vi "File Page - Set Start Trigger.vi"(7 "File Ctl Refs":T3, 8 "error in (no error)":errorcluster, 10 "Start Trigger":T1, 11 "Item Ref in":T2 format="%.0x") -> (0 "error out":errorcluster)   [LabVIEW 2015, in "Waveform Data Logger System Explorer.lvlib"]
uses:
  Waveform Data Logger System Explorer.lvlib
  Types/File Ctl Refs.ctl
  Types/File - Spec Ctl Refs.ctl
  Types/File - Wfm Ctl Refs.ctl
  Types/File - Settings Ctl Refs.ctl
  Shared/Classes/Log File Specifications/Log File Specification/File Conflict Operation.ctl
  Types/File - Start Trig Ctl Refs.ctl
  Shared/Types/Start Trigger.ctl
  Shared/Types/Default Trigger.ctl
  Shared/Types/Digital Trigger.ctl
  Shared/Types/Analog Trigger.ctl
  Shared/Types/In Range Trigger.ctl
  Shared/Types/Value Change Trigger.ctl
  Shared/Types/Boolean Trigger.ctl
  Types/Single Node Browser Data.ctl
  <vilib>/NI Veristand/UI Controls/Single Node Browser/Single Node Browser Ref.ctl
  NationalInstruments.VeriStand.SystemStorageUI
  <vilib>/NI Veristand/UI Controls/Single Node Browser/Callback Type.ctl
  <vilib>/NI Veristand/UI Controls/Single Node Browser/Net Event Data.ctl
  <vilib>/NI Veristand/UI Controls/Single Node Browser/Net Event.ctl
  Types/File - Stop Trig Ctl Refs.ctl
  Shared/Types/Stop Trigger.ctl
  Types/File - Advanced Ctl Refs.ctl
  Types/Log Timestamps.ctl
  <vilib>/NI Veristand/Custom Device API/Custom Device Item Ref.ctl
  NationalInstruments.VeriStand.SystemStorage
  Shared/Globals/Property Strings.vi
  <vilib>/NI Veristand/Custom Device API/Set Item Property (U16).vi
  <vilib>/NI Veristand/Custom Device API/Get Item Property (Dependent Node Pointer).vi
  <vilib>/NI Veristand/Custom Device API/Set Item Property (Dependent Node Pointer).vi
  <vilib>/NI VeriStand/Custom Device API/Custom Device API.lvlib
  Shared/Waveform Data Logger Shared.lvlib
  Shared/Classes/Log File Specifications/Log File Specification/Log File Specification.lvclass
  <vilib>/NI VeriStand/UI Controls/Single Node Browser/NI_VS UI Single Node Browser.lvlib
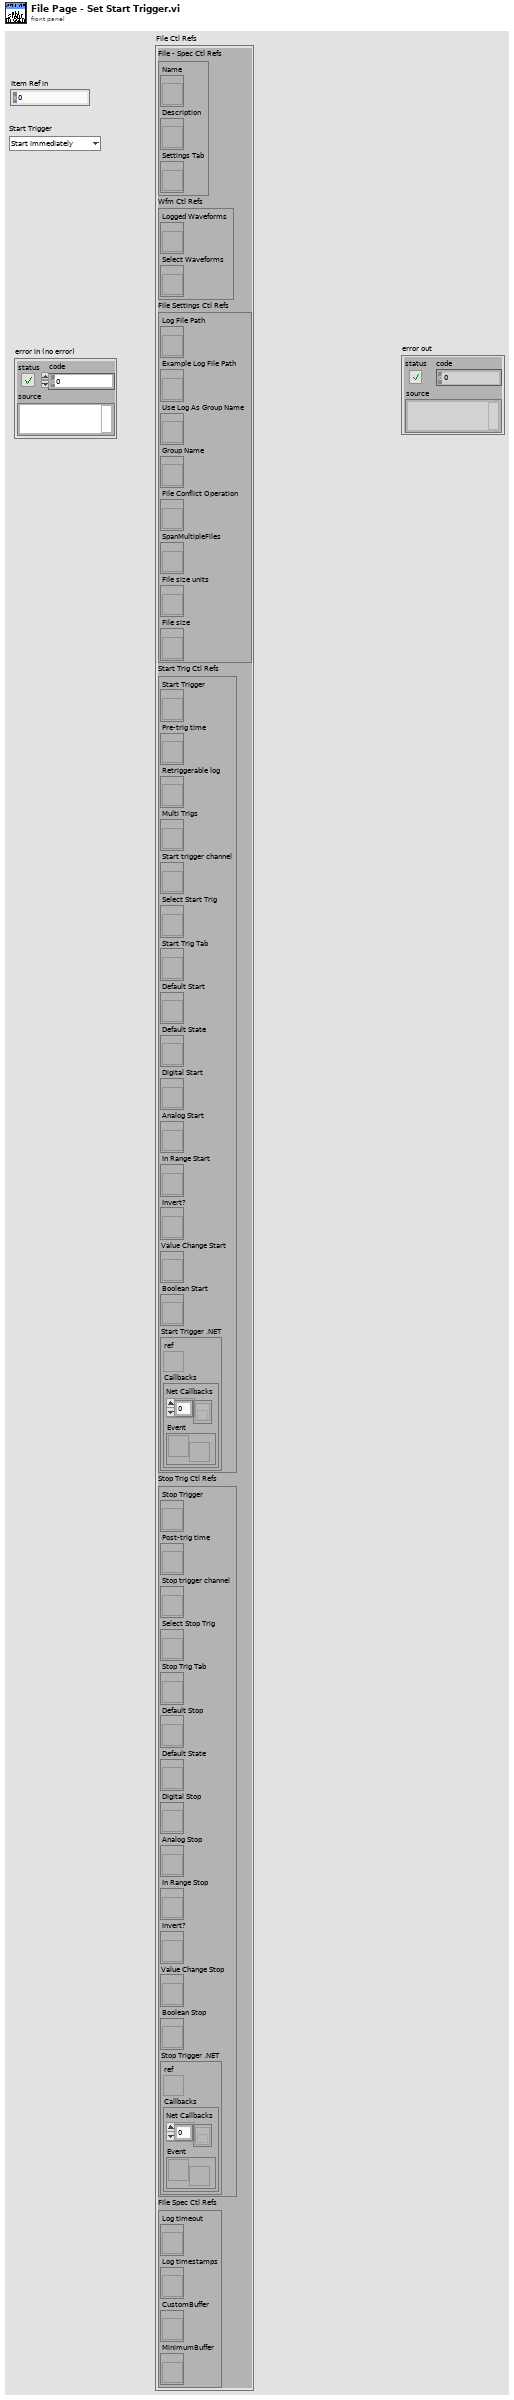
[diagram p1: front panel]
types:
  T1 = typedef "Waveform Data Logger Shared.lvlib/Start Trigger.ctl" = enum16{"Start immediately", "Start on digital edge", "Start on analog edge", "Start when in range", "Start when out of range", "Start on value change", "Start when Boolean condition is true"}
  T2 = typedef "Custom Device API.lvlib/Custom Device Item Ref.ctl" = u64
  T3 = typedef "Waveform Data Logger System Explorer.lvlib/File Ctl Refs.ctl" = cluster{"File Spec Ctl Refs":T4, "Wfm Ctl Refs":T5, "File Settings Ctl Refs":T6, "Start Trig Ctl Refs":T7, "Stop Trig Ctl Refs":T11, "File Spec Ctl Refs":T12}
  T4 = typedef "Waveform Data Logger System Explorer.lvlib/File - Spec Ctl Refs.ctl" = cluster{"Name":refnum<vi>, "Description":refnum<vi>, "Settings Tab":refnum<vi>}
  T5 = typedef "Waveform Data Logger System Explorer.lvlib/File - Wfm Ctl Refs.ctl" = cluster{"Logged Waveforms":refnum<vi>, "Select Waveforms":refnum<vi>}
  T6 = typedef "Waveform Data Logger System Explorer.lvlib/File - Settings Ctl Refs.ctl" = cluster{"Log File Path":refnum<vi>, "Example Log File Path":refnum<vi>, "Use Log As Group Name":refnum<vi>, "Group Name":refnum<vi>, "File Conflict Operation":refnum<vi>, "SpanMultipleFiles":refnum<vi>, "File size units":refnum<vi>, "File size":refnum<vi>}
  T7 = typedef "Waveform Data Logger System Explorer.lvlib/File - Start Trig Ctl Refs.ctl" = cluster{"Start Trigger":refnum<vi>, "Pre-trig time":refnum<vi>, "Retriggerable log":refnum<vi>, "Multi Trigs":refnum<vi>, "Start trigger channel":refnum<vi>, "Select Start Trig":refnum<vi>, "Start Trig Tab":refnum<vi>, "Default Start":refnum<vi>, "Default State":refnum<vi>, "Digital Start":refnum<vi>, "Analog Start":refnum<vi>, "In Range Start":refnum<vi>, "Invert?":refnum<vi>, "Value Change Start":refnum<vi>, "Boolean Start":refnum<vi>, "Start Trigger .NET":T8}
  T8 = typedef "Waveform Data Logger System Explorer.lvlib/Single Node Browser Data.ctl" = cluster{"ref":T9, "Callbacks":T10}
  T9 = typedef "NI_VS UI Single Node Browser.lvlib/Single Node Browser Ref.ctl" = refnum<k24>
  T10 = typedef "NI_VS UI Single Node Browser.lvlib/Callback Type.ctl" = cluster{"Net Callbacks":refnum<k27>[], "Event":refnum<user-event>}
  T11 = typedef "Waveform Data Logger System Explorer.lvlib/File - Stop Trig Ctl Refs.ctl" = cluster{"Stop Trigger":refnum<vi>, "Post-trig time":refnum<vi>, "Stop trigger channel":refnum<vi>, "Select Stop Trig":refnum<vi>, "Stop Trig Tab":refnum<vi>, "Default Stop":refnum<vi>, "Default State":refnum<vi>, "Digital Stop":refnum<vi>, "Analog Stop":refnum<vi>, "In Range Stop":refnum<vi>, "Invert?":refnum<vi>, "Value Change Stop":refnum<vi>, "Boolean Stop":refnum<vi>, "Stop Trigger .NET":T8}
  T12 = typedef "Waveform Data Logger System Explorer.lvlib/File - Advanced Ctl Refs.ctl" = cluster{"Log timeout":refnum<vi>, "Log timestamps":refnum<vi>, "CustomBuffer":refnum<vi>, "MinimumBuffer":refnum<vi>}
  T13 = typedef "Waveform Data Logger Shared.lvlib/Stop Trigger.ctl" = enum16{"Log indefinitely", "Stop after duration", "Stop on digital edge", "Stop on analog edge", "Stop when in range", "Stop when out of range", "Stop on value change", "Stop when Boolean condition is true"}
  T14 = enum32{"Default", "Digital", "Analog", "In Range", "Value Change", "Boolean"}
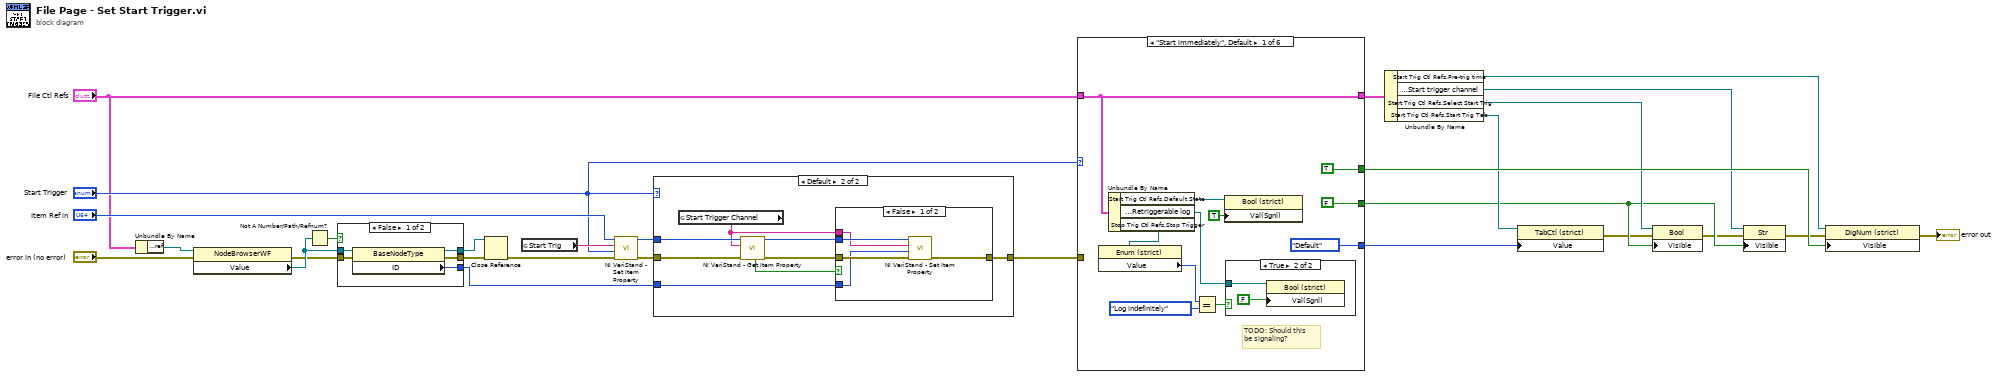
[diagram p0: block diagram]
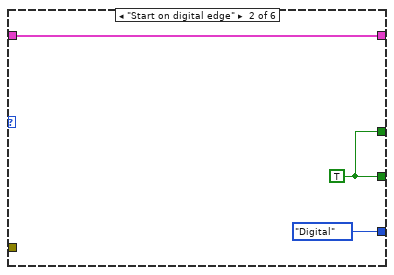
[diagram p3: hidden frame]
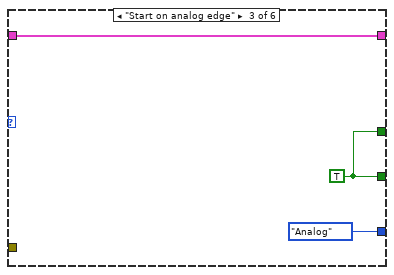
[diagram p4: hidden frame]
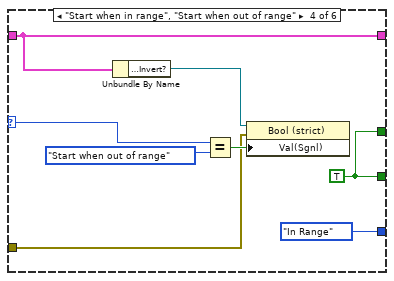
[diagram p5: hidden frame]
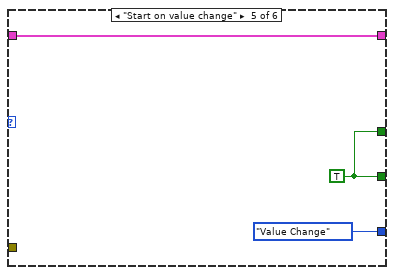
[diagram p6: hidden frame]
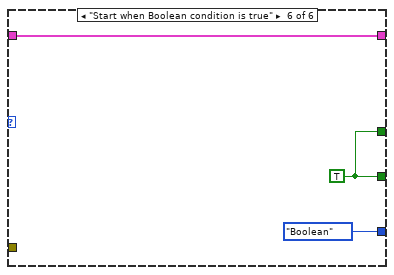
[diagram p7: hidden frame]
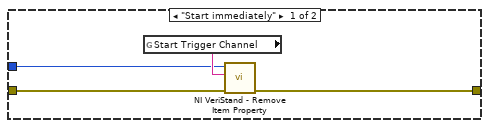
[diagram p8: hidden frame]
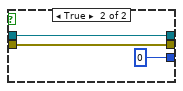
[diagram p10: hidden frame]
diagram:
  n1 = Unbundle By Name("File Ctl Refs") -> ("Start Trig Ctl Refs.Start Trigger .NET.ref"=w27:T9)
  n2 = property class="NodeBrowserWF"(reference=w27, error in="error in (no error)") -> (error out=w24:errorcluster, "Value"=w25:refnum<k24>)  [unwired: 1 out]
  n3 = Not A Number/Path/Refnum?(number/path/refnum=w25) -> (NaN/Path/Refnum?=w26:bool)
  n4 = case shown="False" w26 {
    tunnel: [w33 u64 0 ("ID")] -> w16
    tunnel: w24 -> [w32 w36]
    tunnel: [w29 w36] -> w23
    tunnel: w25 -> [w31 w34]
    tunnel: [w30 w34] -> w22
    frame False {
      n5 = property class="BaseNodeType"(reference=w31, error in=w32) -> (reference out=w30:refnum<k24>, error out=w29:errorcluster, "ID"=w33:u64)
    }
    frame True {
    }
  }
  n6 = Close Reference(reference=w22, error in (no error)=w23) -> (error out=w20:errorcluster)
  n7 = global read "Property Strings.vi" "Start Trig"() -> (w21:string)
  n8 = call-poly <vilib>:"NI VeriStand - Set Item Property.vi"("error in (no error)"=w20, "Value"="Start Trigger", "Property Name"=w21, "Item Ref in"="Item Ref in") -> ("error out"=w17:errorcluster, "Item Ref out"=w18:T2)  [unwired: 5 in, 1 out]
  n9 = case shown="Default" "Start Trigger" {
    tunnel: w17 -> [w39 w46]
    tunnel: w18 -> [w38 w47]
    tunnel: [w37 w48] -> w12
    tunnel: w16 -> [_ w41]
    frame "Start immediately" {
      n10 = global read "Property Strings.vi" "Start Trigger Channel"() -> (w40:string)
      n11 = call <vilib>:"NI VeriStand - Remove Item Property.vi"("error in (no error)"=w39, "Property Name"=w40, "Item Ref in"=w38) -> ("error out"=w37:errorcluster)  [unwired: 6 in, 2 out]
    }
    frame Default {
      n12 = global read "Property Strings.vi" "Start Trigger Channel"() -> (w42:string)
      n13 = call-poly <vilib>:"NI VeriStand - Get Item Property.vi"("error in (no error)"=w46, "Property Name"=w42, "Item Ref in"=w47) -> ("error out"=w44:errorcluster, "Item Ref out"=w43:T2, "Found"=w45:bool)  [unwired: 6 out]
      n14 = case shown="False" w45 {
        tunnel: [w53 w54] -> w48
        tunnel: w44 -> [w52 w54]
        tunnel: w43 -> [w51 _]
        tunnel: w42 -> [w50 _]
        tunnel: w41 -> [w49 _]
        frame False {
          n15 = call-poly <vilib>:"NI VeriStand - Set Item Property.vi"("error in (no error)"=w52, "Dependent Node Ref"=w49, "Property Name"=w50, "Item Ref in"=w51) -> ("error out"=w53:errorcluster)  [unwired: 7 out]
        }
        frame True {
        }
      }
    }
  }
  n16 = case shown="\"Start immediately\", Default" "Start Trigger" {
    selector: "Start Trigger" -> [_ _ _ w80 _ _]
    tunnel: [FALSE w69 w72 w77 w83 w86] -> w7
    tunnel: [T14."Default" ("Start Trig Tab") T14."Digital" ("Start Trig Tab") T14."Analog" ("Start Trig Tab") T14."In Range" ("Start Trig Tab") T14."Value Change" ("Start Trig Tab") T14."Boolean" ("Start Trig Tab")] -> w9
    tunnel: [TRUE w69 w72 w77 w83 w86] -> w15
    tunnel: "File Ctl Refs" -> [w57 w68 w71 w74 w82 w85]
    tunnel: [w57 w68 w71 w74 w82 w85] -> w11
    tunnel: w12 -> [_ _ _ w75 _ _]
    frame "Start immediately", Default {
      # "TODO: Should this\nbe signaling?"
      n17 = Unbundle By Name(w57) -> ("Start Trig Ctl Refs.Default State"=w60:refnum<vi>, "Start Trig Ctl Refs.Retriggerable log"=w58:refnum<vi>, "Stop Trig Ctl Refs.Stop Trigger"=w56:refnum<vi>)
      n18 = property class="Enum (strict)"(reference=w56) -> ("Value"=w55:T13)  [unwired: 1 in, 2 out]
      n19 = Equal?(x=w55, y=Stop_Trigger."Log indefinitely") -> (x = y?=w61:bool)
      n20 = property class="Bool (strict)"(reference=w60, "Val(Sgnl)"=TRUE ("Value (Signaling)")) -> ()  [unwired: 1 in, 2 out]
      n21 = case shown="True" w61 {
        tunnel: w58 -> [_ w66]
        frame False {
        }
        frame True {
          n22 = property on="Property Node" class="Bool (strict)"(reference=w66, "Val(Sgnl)"=FALSE ("Value (Signaling)")) -> ()  [unwired: 1 in, 2 out]
        }
      }
    }
    frame "Start on digital edge" {
      w69 = TRUE
    }
    frame "Start on analog edge" {
      w72 = TRUE
    }
    frame "Start when in range", "Start when out of range" {
      w77 = TRUE
      n23 = Unbundle By Name(w74) -> ("Stop Trig Ctl Refs.Invert?"=w76:refnum<vi>)
      n24 = Equal?(x=w80, y=Start_Trigger."Start when out of range") -> (x = y?=w78:bool)
      n25 = property on="Property Node" class="Bool (strict)"(reference=w76, error in=w75, "Val(Sgnl)"=w78) -> ()  [unwired: 2 out]
    }
    frame "Start on value change" {
      w83 = TRUE
    }
    frame "Start when Boolean condition is true" {
      w86 = TRUE
    }
  }
  n26 = Unbundle By Name(w11) -> ("Start Trig Ctl Refs.Pre-trig time"=w3:refnum<vi>, "Start Trig Ctl Refs.Start trigger channel"=w6:refnum<vi>, "Start Trig Ctl Refs.Select Start Trig"=w8:refnum<vi>, "Start Trig Ctl Refs.Start Trig Tab"=w10:refnum<vi>)
  n27 = property class="TabCtl (strict)"(reference=w10, "Value"=w9) -> (error out=w5:errorcluster)  [unwired: 1 in, 1 out]
  n28 = property class="Bool"(reference=w8, error in=w5, "Visible"=w7) -> (error out=w4:errorcluster)  [unwired: 1 out]
  n29 = property on="Property Node" class="Str"(reference=w6, error in=w4, "Visible"=w7) -> (error out=w2:errorcluster)  [unwired: 1 out]
  n30 = property on="Property Node" class="DigNum (strict)"(reference=w3, error in=w2, "Visible"=w15) -> (error out=→"error out":errorcluster)  [unwired: 1 out]
